vi "Get csv config file data.vi"(8 "error in (no error)":errorcluster, 10 "Filename":string, 11 "Config file":path=path "s:/test/Keyence_sr2000_Scanner/Configs/Keyence_config_table.txt") -> (0 "error out":errorcluster, 1 "Part Number":string, 3 "Line array":string[](array[string]))   [LabVIEW 2013]
panel:
  in  "Edit Config File":bool
  in  "Part Number":i32(listbox)
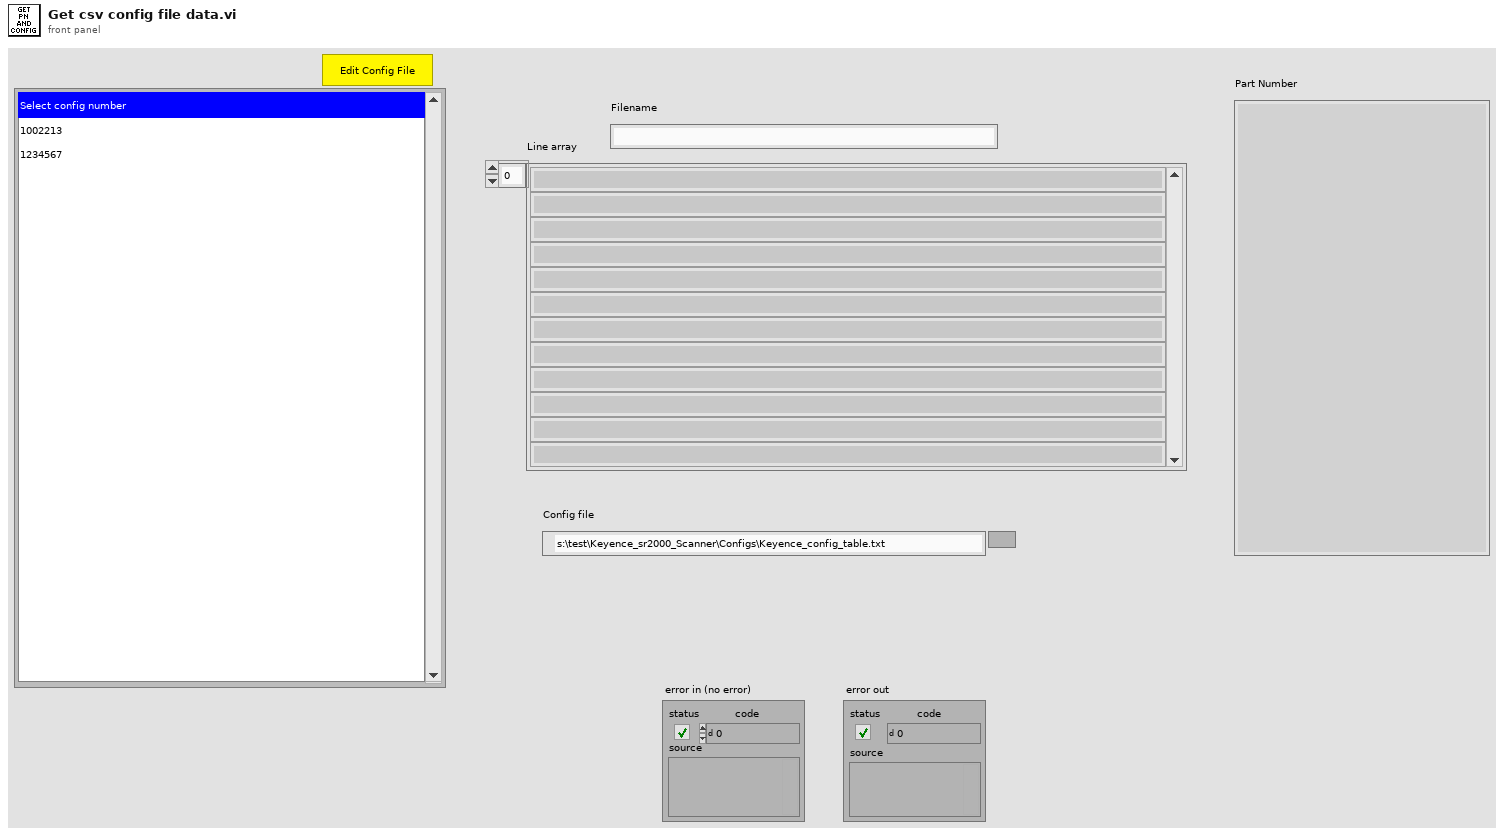
[diagram p1: front panel]
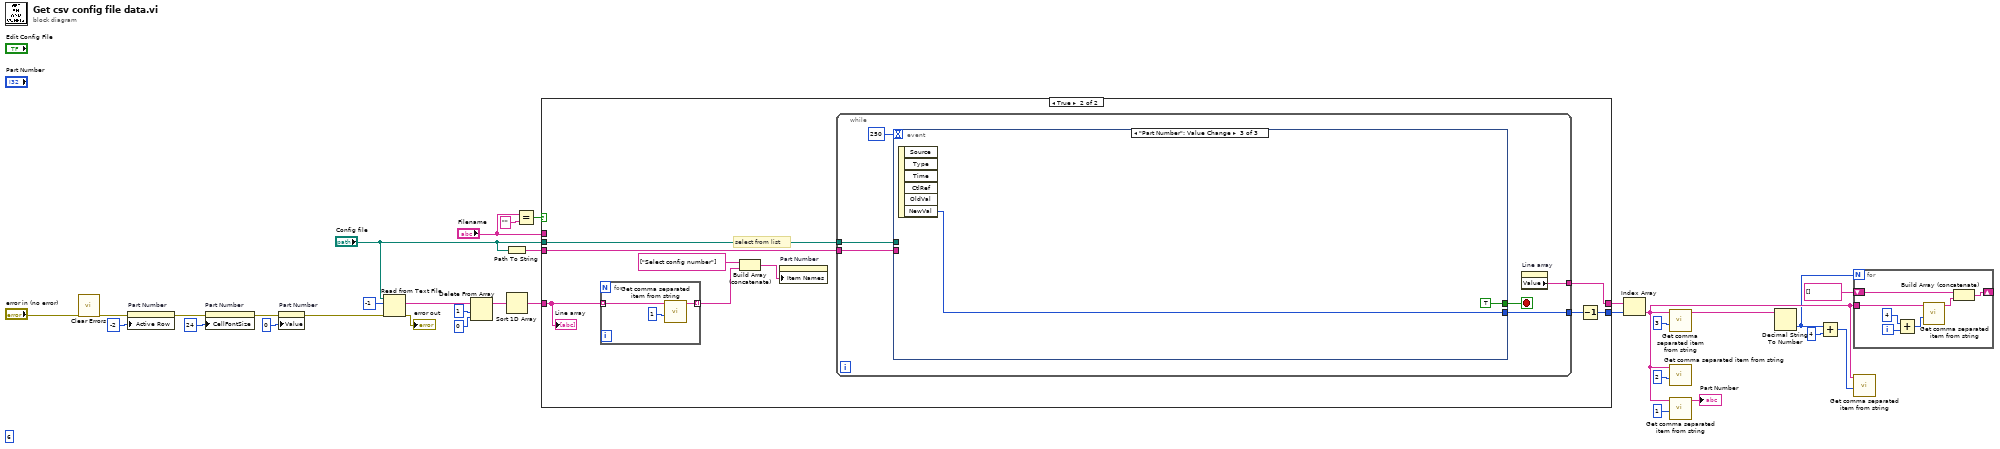
[diagram p0: block diagram]
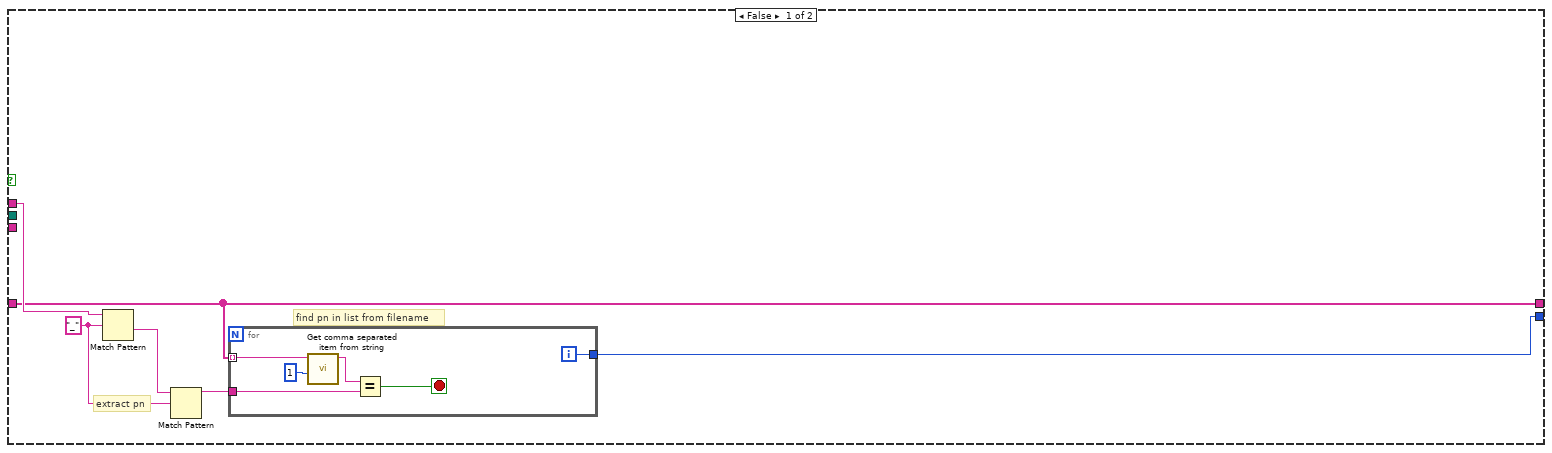
[diagram p2: hidden frame]
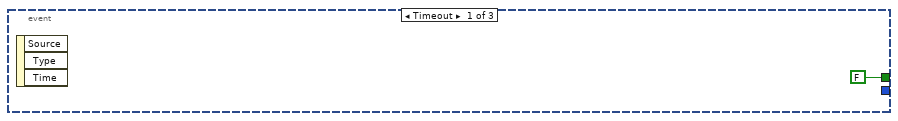
[diagram p3: hidden frame]
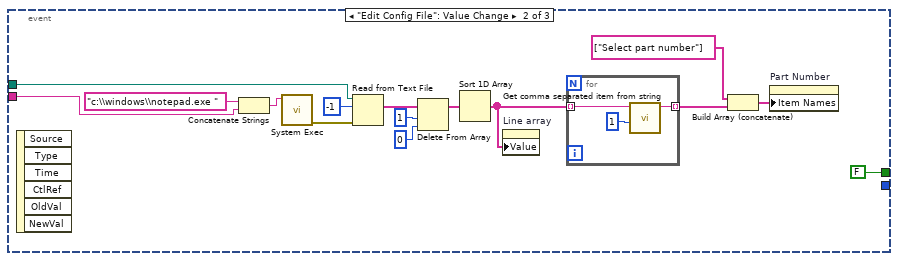
[diagram p4: hidden frame]
diagram:
  (unwired) u32 6 ("Item number")
  n1 = call <vilib>:"Clear Errors.vi"("error in (no error)"="error in (no error)") -> ("error out"=w20:errorcluster)  [unwired: 6 in]
  n2 = property on="Part Number" class="LstBox (strict)"(error in=w20, "Active Row"=-2 ("Active Row:Active Row Number")) -> (error out=w29:errorcluster)  [unwired: 1 in, 1 out]
  n3 = property on="Part Number" class="LstBox (strict)"(error in=w29, "CellFontSize"=u32 24 ("Active Row:Cell Font:Size")) -> (error out=w28:errorcluster)  [unwired: 1 in, 1 out]
  n4 = property on="Part Number" class="LstBox (strict)"(error in=w28, "Value"=0 ("Part Number")) -> (error out=w27:errorcluster)  [unwired: 1 in, 1 out]
  n5 = Read from Text File(file (use dialog)="Config file", count=-1, error in=w27) -> (text=w8:string[], error out=→"error out":errorcluster)  [unwired: 1 in, 2 out]
  n6 = Delete From Array(array=w8, length=1, index=0) -> (array with subset deleted=w5:string[])  [unwired: 1 out]
  n7 = Path To String(path="Config file") -> (string=w3:string)
  n8 = Sort 1D Array(array=w5) -> (sorted array=w4:string[])
  n9 = Equal?(x="Filename", y="") -> (x = y?=w18:bool)
  n10 = case shown="True" w18 {
    tunnel: [w35 w51] -> w22
    tunnel: w4 -> [w34 w48]
    tunnel: "Filename" -> [w39 _]
    tunnel: w3 -> [_ w50]
    tunnel: "Config file" -> [_ w49]
    tunnel: [w34 w46] -> w1
    frame False {
      w37 = "_" ("regular expression")
      # "extract pn"
      # "find pn in list from filename"
      n11 = Match Pattern(string=w39, regular expression=w37) -> (after substring=w38:string)  [unwired: 1 in, 3 out]
      n12 = Match Pattern(string=w38, regular expression=w37) -> (before substring=w36:string)  [unwired: 1 in, 3 out]
      n13 = for {
        tunnel: w34 -> [w44] mode=indexing
        tunnel: w36 -> [w43]
        tunnel: [w40] -> w35
        i -> [w40]
        stop <- w41 stop-if-true
        n14 = call "Get comma separated item from string.vi"("Field Num (1-n)"=u32 1 ("Item number"), "String to parse with commas"=w44) -> ("Item string value"=w42:string)  [unwired: 8 in, 1 out]
        n15 = Equal?(x=w42, y=w43) -> (x = y?=w41:bool)
      }
    }
    frame True {
      # "select from list"
      n16 = for {
        tunnel: w48 -> [w57] mode=indexing
        tunnel: [w55] -> w53 mode=indexing
        n17 = call "Get comma separated item from string.vi"("Field Num (1-n)"=u32 1 ("Item number"), "String to parse with commas"=w57) -> ("Item string value"=w55:string)  [unwired: 8 in, 1 out]
      }
      n18 = Build Array (concatenate)(string[] ["Select config number"] ("Item Names"), w53) -> (w47:string[])
      n19 = property on="Part Number" class="LstBox (strict)"("Item Names"=w47) -> ()  [unwired: 2 in, 2 out]
      n20 = while {
        tunnel: [w61] -> w52
        tunnel: w50 -> [w60]
        tunnel: w49 -> [w59]
        tunnel: [w58] -> w46
        stop <- w63 stop-if-true
        n21 = event shown="[2] \"Part Number\": Value Change" {
          selector: _ -> [_ _ _]
          dyn-events: _ -> [_ _ _]
          timeout: 250 -> [_ _ _]
          tunnel: [FALSE FALSE TRUE] -> w63
          tunnel: [_ _ w83] -> w61
          tunnel: w60 -> [_ w79 _]
          tunnel: w59 -> [_ w75 _]
          event Timeout {
            n22 = event-data() -> ()  [unwired: 1 in, 3 out]
          }
          event "Edit Config File": Value Change {
            n23 = event-data() -> ()  [unwired: 1 in, 6 out]
            n24 = Concatenate Strings("c:\\windows\\notepad.exe " ("command line"), w79) -> (w77:string)
            n25 = call <vilib>:"System Exec.vi"("command line"=w77) -> ("error out"=w74:errorcluster)  [unwired: 7 in, 3 out]
            n26 = Read from Text File(file (use dialog)=w75, count=-1, error in=w74) -> (text=w70:string[])  [unwired: 1 in, 3 out]
            n27 = Delete From Array(array=w70, length=1, index=0) -> (array with subset deleted=w73:string[])  [unwired: 1 out]
            n28 = Sort 1D Array(array=w73) -> (sorted array=w66:string[])
            n29 = property on="Line array" class="Arr (strict)"("Value"=w66) -> ()  [unwired: 2 in, 2 out]
            n30 = for {
              tunnel: w66 -> [w82] mode=indexing
              tunnel: [w80] -> w67 mode=indexing
              n31 = call "Get comma separated item from string.vi"("Field Num (1-n)"=u32 1 ("Item number"), "String to parse with commas"=w82) -> ("Item string value"=w80:string)  [unwired: 8 in, 1 out]
            }
            n32 = Build Array (concatenate)(string[] ["Select part number"] ("Item Names"), w67) -> (w68:string[])
            n33 = property on="Part Number" class="LstBox (strict)"("Item Names"=w68) -> ()  [unwired: 2 in, 2 out]
          }
          event "Part Number": Value Change {
            n34 = event-data() -> ("NewVal"=w83:i32)  [unwired: 1 in, 5 out]
          }
        }
        n35 = property on="Line array" class="Arr (strict)"() -> ("Value"=w58:string[])  [unwired: 2 in, 2 out]
      }
      n36 = Decrement(x=w52) -> (x-1=w51:i32)
      "Line array" <- w48
    }
  }
  n37 = Index Array(array=w1, index=w22) -> (element=w13:string)
  n38 = call "Get comma separated item from string.vi"("Field Num (1-n)"=u32 3 ("Item number"), "String to parse with commas"=w13) -> ("Item string value"=w15:string)  [unwired: 8 in, 1 out]
  n39 = call "Get comma separated item from string.vi"("Field Num (1-n)"=u32 2 ("Item number"), "String to parse with commas"=w13) -> ()  [unwired: 8 in, 2 out]
  n40 = call "Get comma separated item from string.vi"("Field Num (1-n)"=u32 1 ("Item number"), "String to parse with commas"=w13) -> ("Item string value"=→"Part Number":string)  [unwired: 8 in, 1 out]
  n41 = Decimal String To Number(string=w15) -> (number=w10:i32)  [unwired: 2 in, 1 out]
  n42 = Add(x=w10, y=u32 4 ("Item number")) -> (x+y=w9:u32)
  n43 = for {
    N: w10 -> [_]
    tunnel: w13 -> [w91]
    shift-right: [w85] -> w12
    shift-left: string[] [] -> [w87]
    i -> [w90]
    n44 = Add(x=4, y=w90) -> (x+y=w88:i32)
    n45 = call "Get comma separated item from string.vi"("Field Num (1-n)"=w88, "String to parse with commas"=w91) -> ("Item string value"=w86:string)  [unwired: 8 in, 1 out]
    n46 = Build Array (concatenate)(w87, w86) -> (w85:string[])
  }
  n47 = call "Get comma separated item from string.vi"("Field Num (1-n)"=w9, "String to parse with commas"=w13) -> ()  [unwired: 8 in, 2 out]
